vi "eFGV - Trigger Alarm.vi"(6 "States":T2, 8 "Error In":errorcluster, 11 "Alarm Trigger Data":T1) -> (0 "Error Out":errorcluster, 2 "Alarm Trigger Data 2":refnum<user-event>)   [LabVIEW 2020]
uses:
  Control/State - eFGV.ctl
  Control/Alarm Trigger Data.ctl
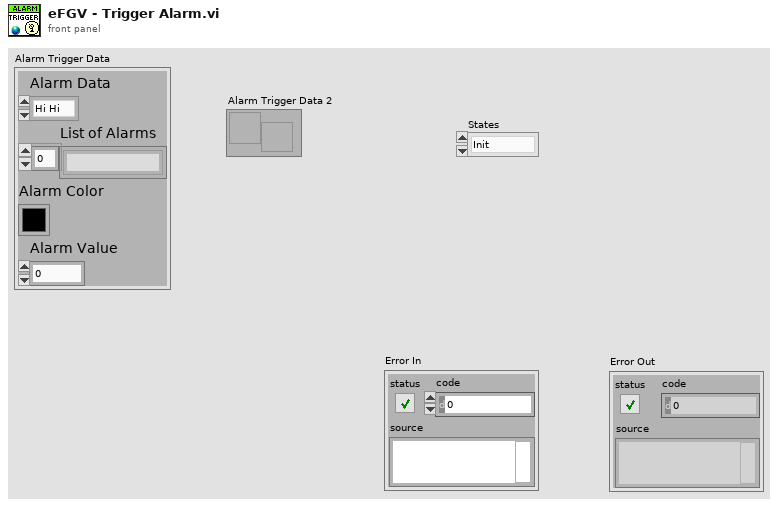
[diagram p1: front panel]
types:
  T1 = typedef "Alarm Trigger Data.ctl" = cluster{"Alarm Data":enum16{"Hi Hi", "Hi", "OK", "Lo", "Lo Lo"}, "List of Alarms":string[], "Alarm Color":u32, "Alarm Value":dbl}
  T2 = typedef "State - eFGV.ctl" = enum16{"Init", "Read", "Write", "Exit"}
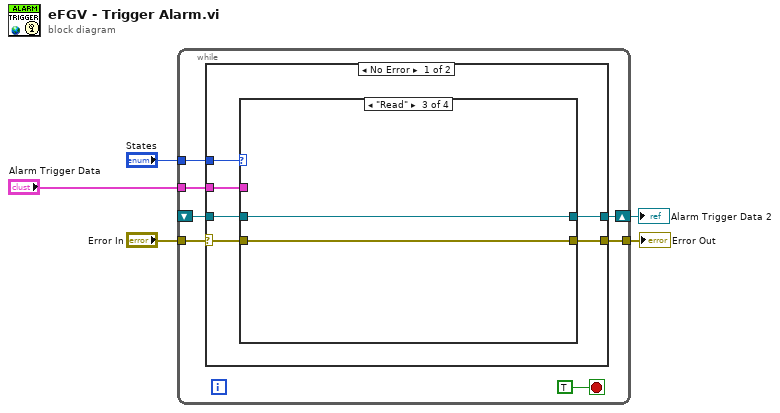
[diagram p0: block diagram]
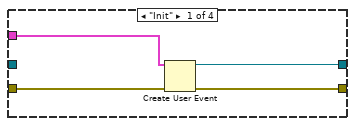
[diagram p2: hidden frame]
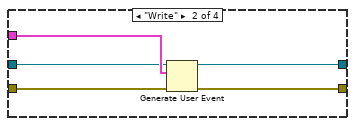
[diagram p3: hidden frame]
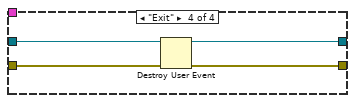
[diagram p4: hidden frame]
diagram:
  n1 = while {
    tunnel: "Error In" -> [w11]
    tunnel: [w10] -> w4
    tunnel: "States" -> [w9]
    shift-right: [w8] -> w1
    shift-left: _ -> [w7]
    tunnel: "Alarm Trigger Data" -> [w6]
    stop <- TRUE stop-if-true
    n2 = case shown="No Error" w11 {
      selector: w11 -> [w17 w34]
      tunnel: [w16 w34] -> w10
      tunnel: w9 -> [w18 _]
      tunnel: [w15 w33] -> w8
      tunnel: w7 -> [w14 w33]
      tunnel: w6 -> [w13 _]
      frame No Error {
        n3 = case shown="\"Read\"" w18 {
          tunnel: w17 -> [w22 w27 w29 w32]
          tunnel: [w21 w26 w29 w31] -> w16
          tunnel: [w19 w24 w28 w30] -> w15
          tunnel: w14 -> [_ w23 w28 w30]
          tunnel: w13 -> [w20 w25 _ _]
          frame "Init" {
            n4 = Create User Event(user event datatype=w20, error in=w22) -> (user event=w19:refnum<user-event>, error out=w21:errorcluster)
          }
          frame "Write" {
            n5 = Generate User Event(user event=w23, event data cluster=w25, error in=w27) -> (user event out=w24:refnum<user-event>, error out=w26:errorcluster)  [unwired: 1 in]
          }
          frame "Read" {
          }
          frame "Exit" {
            n6 = Destroy User Event(user event=w30, error in=w32) -> (error out=w31:errorcluster)
          }
        }
      }
      frame Error {
      }
    }
  }
  "Error Out" <- w4
  "Alarm Trigger Data 2" <- w1
